vi "FTW-JSON-LexicalScan-IsControlChar.vi"(0 "Lex In":T1, 11 "error in (no error)":errorcluster) -> (4 "Lex Out":T1, 15 "error out":errorcluster)   [LabVIEW 2015]
uses:
  FTW-JSON-LexicalScan.ctl
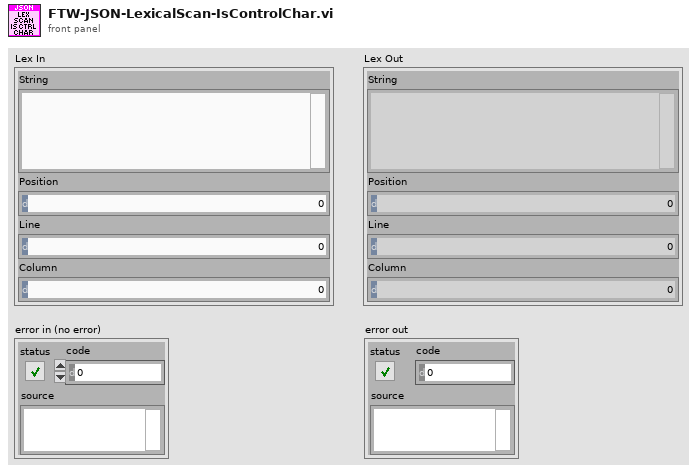
[diagram p1: front panel]
types:
  T1 = typedef "FTW-JSON-LexicalScan.ctl" = cluster{"String":string, "Position":i32, "Line":i32, "Column":i32}
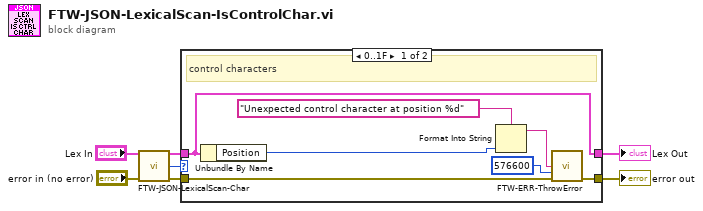
[diagram p0: block diagram]
diagram:
  n1 = call "FTW-JSON-LexicalScan-Char.vi"("JSON String"="Lex In", "error in"="error in (no error)") -> ("JSON String Out"=w5:T1, "Char"=w6:u8, "error out"=w7:errorcluster)  [unwired: 11 in]
  n2 = case shown="0..1F" w6 {
    tunnel: w5 -> [w8 w15]
    tunnel: w7 -> [w10 w16]
    tunnel: [w9 w16] -> w1
    tunnel: [w8 w15] -> w2
    frame 0..31 {
      # "control characters"
      n3 = Unbundle By Name(w8) -> ("Position"=w12:i32)
      n4 = Format Into String(format string="Unexpected control character at position %d" ("Error Message"), w12) -> (resulting string=w13:string)  [unwired: 2 in, 1 out]
      n5 = call "FTW-ERR-ThrowError.vi"("Error Message"=w13, "Error Code"=576600, "error in"=w10) -> ("error out"=w9:errorcluster)  [unwired: 12 in]
    }
    frame Default {
      # "any unicode except control char"
    }
  }
  "error out" <- w1
  "Lex Out" <- w2
